vi "rsidr_core_global.vi"() -> ()   [LabVIEW 2020, in "Rohde&Schwarz RTx Oscilloscopes.lvlib"] (continued)
"Descriptive Name"="Protocol SPI Frame Data MOSI", "Data Type"=2, "Command"="BUS{SerialBus}:SPI:FRAM<Frame>:DATA:MOSI?", "Access"=0, "Range Table"="", "Read Callback"="rsrtx_FormatSPIFrameRepCapString_ReadCallback.vi", "Write Callback"="", "Supported Models"="", "Instrument Options"="", "Flags"=0, "Help"="Returns the data words of the specified frame of the MOSI line.\n\nAvailable Repeated Capabilities:\nSerialBus: SB1, SB2, SB3, SB4\r\n\nRemote-control command(s):\nBUS<b>:SPI:FRAMe<n>:DATA:MOSI?"}, {"Level"=3, "Class Only"=FALSE, "Identifier"="RSRTX_ATTR_PROTOCOL_SPI_FRAME_DATA_MISO", "Descriptive Name"="Protocol SPI Frame Data MISO", "Data Type"=2, "Command"="BUS{SerialBus}:SPI:FRAM<Frame>:DATA:MISO?", "Access"=0, "Range Table"="", "Read Callback"="rsrtx_FormatSPIFrameRepCapString_ReadCallback.vi", "Write Callback"="", "Supported Models"="", "Instrument Options"="", "Flags"=0, "Help"="Returns the data words of the specified frame of the MISO line.\n\nAvailable Repeated Capabilities:\nSerialBus: SB1, SB2, SB3, SB4\r\n\nRemote-control command(s):\nBUS<b>:SPI:FRAMe<n>:DATA:MISO?"}, {"Level"=3, "Class Only"=FALSE, "Identifier"="RSRTX_ATTR_PROTOCOL_SPI_WORD_COUNT", "Descriptive Name"="Protocol SPI Word Count", "Data Type"=0, "Command"="BUS{SerialBus}:SPI:FRAM<Frame>:WCO?", "Access"=0, "Range Table"="", "Read Callback"="rsrtx_FormatSPIFrameRepCapInt_ReadCallback.vi", "Write Callback"="", "Supported Models"="", "Instrument Options"="", "Flags"=0, "Help"="Returns the number of words in the specified frame.\n\nAvailable Repeated Capabilities:\nSerialBus: SB1, SB2, SB3, SB4\r\n\nRemote-control command(s):\nBUS<b>:SPI:FRAMe<n>:WCOunt?"}, {"Level"=3, "Class Only"=FALSE, "Identifier"="RSRTX_ATTR_PROTOCOL_SPI_SELECTED_WORD", "Descriptive Name"="Protocol SPI Selected Word", "Data Type"=0, "Command"="", "Access"=2, "Range Table"="", "Read Callback"="", "Write Callback"="", "Supported Models"="", "Instrument Options"="", "Flags"=0, "Help"="Sets selector repeated capability Word.\n\nAvailable Repeated Capabilities:\nNone\n\nRemote-control command(s):\n"}, {"Level"=3, "Class Only"=FALSE, "Identifier"="RSRTX_ATTR_PROTOCOL_SPI_WORD_START", "Descriptive Name"="Protocol SPI Word Start", "Data Type"=1, "Command"="BUS{SerialBus}:SPI:FRAM<Frame>:WORD<Word>:STAR?", "Access"=0, "Range Table"="", "Read Callback"="rsrtx_FormatSPIFrameWordRepCapReal_ReadCallback.vi", "Write Callback"="", "Supported Models"="", "Instrument Options"="", "Flags"=0, "Help"="Returns the start time of the specified data word.\n\nAvailable Repeated Capabilities:\nSerialBus: SB1, SB2, SB3, SB4\r\n\nRemote-control command(s):\nBUS<b>:SPI:FRAMe<n>:WORD<o>:STARt?"}, {"Level"=3, "Class Only"=FALSE, "Identifier"="RSRTX_ATTR_PROTOCOL_SPI_WORD_END", "Descriptive Name"="Protocol SPI Word End", "Data Type"=1, "Command"="BUS{SerialBus}:SPI:FRAM<Frame>:WORD<Word>:STOP?", "Access"=0, "Range Table"="", "Read Callback"="rsrtx_FormatSPIFrameWordRepCapReal_ReadCallback.vi", "Write Callback"="", "Supported Models"="", "Instrument Options"="", "Flags"=0, "Help"="Returns the end time of the specified data word.\n\nAvailable Repeated Capabilities:\nSerialBus: SB1, SB2, SB3, SB4\r\n\nRemote-control command(s):\nBUS<b>:SPI:FRAMe<n>:WORD<o>:STOP?"}, {"Level"=3, "Class Only"=FALSE, "Identifier"="RSRTX_ATTR_PROTOCOL_SPI_WORD_MOSI", "Descriptive Name"="Protocol SPI Word MOSI", "Data Type"=0, "Command"="BUS{SerialBus}:SPI:FRAM<Frame>:WORD<Word>:MOSI?", "Access"=0, "Range Table"="", "Read Callback"="rsrtx_FormatSPIFrameWordRepCapInt_ReadCallback.vi", "Write Callback"="", "Supported Models"="", "Instrument Options"="", "Flags"=0, "Help"="Returns the data value of the specified word on the MOSI line.\nUse this command if only one line is defined.\n\nAvailable Repeated Capabilities:\nSerialBus: SB1, SB2, SB3, SB4\r\n\nRemote-control command(s):\nBUS<b>:SPI:FRAMe<n>:WORD<o>:MOSI?"}, {"Level"=3, "Class Only"=FALSE, "Identifier"="RSRTX_ATTR_PROTOCOL_SPI_WORD_MISO", "Descriptive Name"="Protocol SPI Word MISO", "Data Type"=0, "Command"="BUS{SerialBus}:SPI:FRAM<Frame>:WORD<Word>:MISO?", "Access"=0, "Range Table"="", "Read Callback"="rsrtx_FormatSPIFrameWordRepCapInt_ReadCallback.vi", "Write Callback"="", "Supported Models"="", "Instrument Options"="", "Flags"=0, "Help"="Returns the data value of the specified word on the MISO line.\n\nAvailable Repeated Capabilities:\nSerialBus: SB1, SB2, SB3, SB4\r\n\nRemote-control command(s):\nBUS<b>:SPI:FRAMe<n>:WORD<o>:MISO?"}, {"Level"=3, "Class Only"=TRUE, "Identifier"="", "Descriptive Name"="SSPI", "Data Type"=0, "Command"="", "Access"=0, "Range Table"="", "Read Callback"="", "Write Callback"="", "Supported Models"="", "Instrument Options"="", "Flags"=0, "Help"="SSPI Protocol settings."}, {"Level"=4, "Class Only"=FALSE, "Identifier"="RSRTX_ATTR_PROTOCOL_SSPI_CLOCK_SOURCE", "Descriptive Name"="Protocol SSPI Clock Source", "Data Type"=0, "Command"="BUS{SerialBus}:SSPI:CLOC:SOUR", "Access"=2, "Range Table"="RsRtx_rngChannelAndDigitalSource", "Read Callback"="", "Write Callback"="", "Supported Models"="", "Instrument Options"="", "Flags"=0, "Help"="Sets the input channel for the clock lines.\n\nAvailable Repeated Capabilities:\nSerialBus: SB1, SB2, SB3, SB4\r\n\nRemote-control command(s):\nBUS<b>:SSPI:CLOCk:SOURce"}, {"Level"=4, "Class Only"=FALSE, "Identifier"="RSRTX_ATTR_PROTOCOL_SSPI_DATA_SOURCE", "Descriptive Name"="Protocol SSPI Data Source", "Data Type"=0, "Command"="BUS{SerialBus}:SSPI:DATA:SOUR", "Access"=2, "Range Table"="rsrtx_rngMOSISource", "Read Callback"="", "Write Callback"="", "Supported Models"="", "Instrument Options"="", "Flags"=0, "Help"="Sets the input channel for the clock lines.\n\nAvailable Repeated Capabilities:\nSerialBus: SB1, SB2, SB3, SB4\r\n\nRemote-control command(s):\nBUS<b>:SSPI:DATA:SOURce"}, {"Level"=4, "Class Only"=FALSE, "Identifier"="RSRTX_ATTR_PROTOCOL_SSPI_MISO_SOURCE", "Descriptive Name"="Protocol SSPI MISO Source", "Data Type"=0, "Command"="BUS{SerialBus}:SSPI:MISO:SOUR", "Access"=2, "Range Table"="rsrtx_rngMISOSource", "Read Callback"="", "Write Callback"="", "Supported Models"="", "Instrument Options"="", "Flags"=0, "Help"="Selects the input channel of the optional MISO line.\n\nAvailable Repeated Capabilities:\nSerialBus: SB1, SB2, SB3, SB4\r\n\nRemote-control command(s):\nBUS<b>:SSPI:MISO:SOURce"}, {"Level"=4, "Class Only"=FALSE, "Identifier"="RSRTX_ATTR_PROTOCOL_SSPI_CLOCK_POLARITY", "Descriptive Name"="Protocol SSPI Clock Polarity", "Data Type"=0, "Command"="BUS{SerialBus}:SSPI:CLOC:POL", "Access"=2, "Range Table"="rsrtx_rngPolarity", "Read Callback"="", "Write Callback"="", "Supported Models"="", "Instrument Options"="", "Flags"=0, "Help"="Selects whether transmitted data is high active (high = 1, Positive) or low active (low = 1, Negative).\n\nAvailable Repeated Capabilities:\nSerialBus: SB1, SB2, SB3, SB4\r\n\nRemote-control command(s):\nBUS<b>:SSPI:CLOCk:POLarity"}, {"Level"=4, "Class Only"=FALSE, "Identifier"="RSRTX_ATTR_PROTOCOL_SSPI_DATA_POLARITY", "Descriptive Name"="Protocol SSPI Data Polarity", "Data Type"=0, "Command"="BUS{SerialBus}:SSPI:DATA:POL", "Access"=2, "Range Table"="rsrtx_rngPolarity", "Read Callback"="", "Write Callback"="", "Supported Models"="", "Instrument Options"="", "Flags"=0, "Help"="Selects whether transmitted data is high active (high = 1, Positive) or low active (low = 1, Negative).\n\nAvailable Repeated Capabilities:\nSerialBus: SB1, SB2, SB3, SB4\r\n\nRemote-control command(s):\nBUS<b>:SSPI:DATA:POLarity"}, {"Level"=4, "Class Only"=FALSE, "Identifier"="RSRTX_ATTR_PROTOCOL_SSPI_INTERFRAME_TIME", "Descriptive Name"="Protocol SSPI Interframe Time", "Data Type"=1, "Command"="BUS{SerialBus}:SSPI:BIT", "Access"=2, "Range Table"="rsrtx_rngProtocolBurstIdleTime", "Read Callback"="", "Write Callback"="", "Supported Models"="", "Instrument Options"="", "Flags"=0, "Help"="Within the idle time the data and clock lines are low. A new frame begins when the idle time has expired and the clock line has been inactive during that time. If the time interval between the data words is shorter than the idle time, the words are part of the same frame.\n\nAvailable Repeated Capabilities:\nSerialBus: SB1, SB2, SB3, SB4\r\n\nRemote-control command(s):\nBUS<b>:SSPI:BITime"}, {"Level"=4, "Class Only"=FALSE, "Identifier"="RSRTX_ATTR_PROTOCOL_SSPI_BIT_ORDER", "Descriptive Name"="Protocol SSPI Bit Order", "Data Type"=0, "Command"="BUS{SerialBus}:SSPI:BORD", "Access"=2, "Range Table"="rsrtx_rngProtocolSPIBitOrder", "Read Callback"="", "Write Callback"="", "Supported Models"="", "Instrument Options"="", "Flags"=0, "Help"="Defines if the data of the messages starts with MSB (most significant bit) or LSB (least significant bit).\n\nAvailable Repeated Capabilities:\nSerialBus: SB1, SB2, SB3, SB4\r\n\nRemote-control command(s):\nBUS<b>:SSPI:BORDer"}, {"Level"=4, "Class Only"=FALSE, "Identifier"="RSRTX_ATTR_PROTOCOL_SSPI_WORD_LENGTH", "Descriptive Name"="Protocol SSPI Word Length", "Data Type"=0, "Command"="BUS{SerialBus}:SSPI:SSIZ", "Access"=2, "Range Table"="rsrtx_rngProtocolSPIWordLength", "Read Callback"="", "Write Callback"="", "Supported Models"="", "Instrument Options"="", "Flags"=0, "Help"="Sets the word length, the number of bits in a message.\n\nAvailable Repeated Capabilities:\nSerialBus: SB1, SB2, SB3, SB4\r\n\nRemote-control command(s):\nBUS<b>:SSPI:SSIZe"}, {"Level"=4, "Class Only"=FALSE, "Identifier"="RSRTX_ATTR_PROTOCOL_SSPI_MOSI_POLARITY", "Descriptive Name"="Protocol SSPI MOSI Polarity", "Data Type"=0, "Command"="BUS{SerialBus}:SSPI:MOSI:POL", "Access"=2, "Range Table"="rsrtx_rngProtocolSPIMISOPolarity", "Read Callback"="", "Write Callback"="", "Supported Models"="", "Instrument Options"="", "Flags"=0, "Help"="Selects if transmitted data is high active (high = 1) or low active (low = 1) on the MOSI/MISO line.\n\nAvailable Repeated Capabilities:\nSerialBus: SB1, SB2, SB3, SB4\r\n\nRemote-control command(s):\nBUS<b>:SSPI:MOSI:POLarity"}, {"Level"=4, "Class Only"=FALSE, "Identifier"="RSRTX_ATTR_PROTOCOL_SSPI_MISO_POLARITY", "Descriptive Name"="Protocol SSPI MISO Polarity", "Data Type"=0, "Command"="BUS{SerialBus}:SSPI:MISO:POL", "Access"=2, "Range Table"="rsrtx_rngProtocolSPIMISOPolarity", "Read Callback"="", "Write Callback"="", "Supported Models"="", "Instrument Options"="", "Flags"=0, "Help"="Selects whether transmitted data is high active (high = 1) or low active (low = 1) on the MISO line.\n\nAvailable Repeated Capabilities:\nSerialBus: SB1, SB2, SB3, SB4\r\n\nRemote-control command(s):\nBUS<b>:SSPI:MISO:POLarity"}, {"Level"=2, "Class Only"=TRUE, "Identifier"="", "Descriptive Name"="UART", "Data Type"=0, "Command"="", "Access"=0, "Range Table"="", "Read Callback"="", "Write Callback"="", "Supported Models"="", "Instrument Options"="", "Flags"=0, "Help"="UART/RS232 (EIA-232 serial interface) - decoding requires option K2"}, {"Level"=3, "Class Only"=FALSE, "Identifier"="RSRTX_ATTR_PROTOCOL_UART_SOURCE", "Descriptive Name"="Protocol UART Source", "Data Type"=0, "Command"="BUS{SerialBus}:UART:DATA:SOUR", "Access"=2, "Range Table"="rsrtx_rngUARTSource", "Read Callback"="", "Write Callback"="", "Supported Models"="", "Instrument Options"="", "Flags"=0, "Help"="Selects the input channel of the UART signal.\n\nAvailable Repeated Capabilities:\nSerialBus: SB1, SB2, SB3, SB4\r\n\nRemote-control command(s):\nBUS<b>:UART:DATA:SOURce"}, {"Level"=3, "Class Only"=FALSE, "Identifier"="RSRTX_ATTR_PROTOCOL_UART_RX_SOURCE_LINE", "Descriptive Name"="Protocol UART RX Source Line", "Data Type"=0, "Command"="BUS{SerialBus}:UART:RX:SOUR", "Access"=2, "Range Table"="rsrtx_rngUARTSource", "Read Callback"="", "Write Callback"="", "Supported Models"="", "Instrument Options"="K2", "Flags"=0, "Help"="Selects the input channel of the UART signal.\n\nAvailable Repeated Capabilities:\nSerialBus: SB1, SB2, SB3, SB4\r\n\nRemote-control command(s):\nBUS<b>:UART:RX:SOURce"}, {"Level"=3, "Class Only"=FALSE, "Identifier"="RSRTX_ATTR_PROTOCOL_UART_TX_SOURCE_LINE", "Descriptive Name"="Protocol UART TX Source Line", "Data Type"=0, "Command"="BUS{SerialBus}:UART:TX:SOUR", "Access"=2, "Range Table"="rsrtx_rngUARTTxSource", "Read Callback"="", "Write Callback"="", "Supported Models"="", "Instrument Options"="K2", "Flags"=0, "Help"="Selects the input channel of the UART signal.\n\nAvailable Repeated Capabilities:\nSerialBus: SB1, SB2, SB3, SB4\r\n\nRemote-control command(s):\nBUS<b>:UART:TX:SOURce"}, {"Level"=3, "Class Only"=FALSE, "Identifier"="RSRTX_ATTR_PROTOCOL_UART_POLARITY", "Descriptive Name"="Protocol UART Polarity", "Data Type"=0, "Command"="BUS{SerialBus}:UART:DATA:POL", "Access"=2, "Range Table"="rsrtx_rngPolarity", "Read Callback"="", "Write Callback"="", "Supported Models"="", "Instrument Options"="", "Flags"=0, "Help"="Selects whether transmitted data is high active (high = 1, Positive) or low active (low = 1, Negative). Alternative Command for RSRTX_ATTR_PROTOCOL_UART_IDLE_STATE_POLARITY.\n\nAvailable Repeated Capabilities:\nSerialBus: SB1, SB2, SB3, SB4\r\n\nRemote-control command(s):\nBUS<b>:UART:DATA:POLarity"}, {"Level"=3, "Class Only"=FALSE, "Identifier"="RSRTX_ATTR_PROTOCOL_UART_IDLE_STATE_POLARITY", "Descriptive Name"="Protocol UART Idle State Polarity", "Data Type"=0, "Command"="BUS{SerialBus}:UART:POL", "Access"=2, "Range Table"="RsRtx_rngIdleStatePolarity", "Read Callback"="", "Write Callback"="", "Supported Models"="", "Instrument Options"="", "Flags"=0, "Help"="Defines the logic levels of the bus. The idle state corresponds to a logic 1, and the start bit to a logic 0.\nAlternative command for RSRTX_ATTR_PROTOCOL_UART_POLARITY\n\nAvailable Repeated Capabilities:\nSerialBus: SB1, SB2, SB3, SB4\r\n\nRemote-control command(s):\nBUS<b>:UART:POLarity"}, {"Level"=3, "Class Only"=FALSE, "Identifier"="RSRTX_ATTR_PROTOCOL_UART_INTERFRAME_TIME", "Descriptive Name"="Protocol UART Interframe Time", "Data Type"=1, "Command"="BUS{SerialBus}:UART:BIT", "Access"=2, "Range Table"="", "Read Callback"="", "Write Callback"="", "Supported Models"="", "Instrument Options"="", "Flags"=0, "Help"="Sets the minimal time between two data frames (packets), that is, between the last stop bit and the start bit of the next frame.\n\nAvailable Repeated Capabilities:\nSerialBus: SB1, SB2, SB3, SB4\r\n\nRemote-control command(s):\nBUS<b>:UART:BITime"}, {"Level"=3, "Class Only"=FALSE, "Identifier"="RSRTX_ATTR_PROTOCOL_UART_WORD_LENGTH", "Descriptive Name"="Protocol UART Word Length", "Data Type"=0, "Command"="BUS{SerialBus}:UART:SSIZ", "Access"=2, "Range Table"="rsrtx_rngProtocolUARTWordLength", "Read Callback"="", "Write Callback"="", "Supported Models"="", "Instrument Options"="", "Flags"=0, "Help"="Sets the number of data bits in a message.\n\nAvailable Repeated Capabilities:\nSerialBus: SB1, SB2, SB3, SB4\r\n\nRemote-control command(s):\nBUS<b>:UART:SSIZe"}, {"Level"=3, "Class Only"=FALSE, "Identifier"="RSRTX_ATTR_PROTOCOL_UART_BIT_RATE", "Descriptive Name"="Protocol UART Bit Rate", "Data Type"=1, "Command"="BUS{SerialBus}:UART:BAUD", "Access"=2, "Range Table"="rsrtx_rngProtocolUARTBitRate", "Read Callback"="", "Write Callback"="", "Supported Models"="", "Instrument Options"="", "Flags"=0, "Help"="Sets the number of transmitted bits per second.\n\nAvailable Repeated Capabilities:\nSerialBus: SB1, SB2, SB3, SB4\r\n\nRemote-control command(s):\nBUS<b>:UART:BAUDrate"}, {"Level"=3, "Class Only"=FALSE, "Identifier"="RSRTX_ATTR_PROTOCOL_UART_PARITY", "Descriptive Name"="Protocol UART Parity", "Data Type"=0, "Command"="BUS{SerialBus}:UART:PAR", "Access"=2, "Range Table"="rsrtx_rngProtocolUARTParity", "Read Callback"="", "Write Callback"="", "Supported Models"="", "Instrument Options"="", "Flags"=0, "Help"="Defines the optional parity bit that is used for error detection.\n\nAvailable Repeated Capabilities:\nSerialBus: SB1, SB2, SB3, SB4\r\n\nRemote-control command(s):\nBUS<b>:UART:PARity"}, {"Level"=3, "Class Only"=FALSE, "Identifier"="RSRTX_ATTR_PROTOCOL_UART_STOP_BITS", "Descriptive Name"="Protocol UART Stop Bits", "Data Type"=0, "Command"="BUS{SerialBus}:UART:SBIT", "Access"=2, "Range Table"="rsrtx_rngProtocolUARTStopBits", "Read Callback"="", "Write Callback"="", "Supported Models"="", "Instrument Options"="", "Flags"=0, "Help"="Sets the stop bits.\n\nAvailable Repeated Capabilities:\nSerialBus: SB1, SB2, SB3, SB4\r\n\nRemote-control command(s):\nBUS<b>:UART:SBIT"}, {"Level"=3, "Class Only"=FALSE, "Identifier"="RSRTX_ATTR_PROTOCOL_UART_FRAME_COUNT", "Descriptive Name"="Protocol UART Frame Count", "Data Type"=0, "Command"="BUS{SerialBus}:UART:FCO?", "Access"=0, "Range Table"="", "Read Callback"="", "Write Callback"="", "Supported Models"="", "Instrument Options"="K2", "Flags"=0, "Help"="Return the number of decoded frames on the data line.\n\nAvailable Repeated Capabilities:\nSerialBus: SB1, SB2, SB3, SB4\r\n\nRemote-control command(s):\nBUS<b>:UART:FCOunt?"}, {"Level"=3, "Class Only"=FALSE, "Identifier"="RSRTX_ATTR_PROTOCOL_UART_RX_FRAME_COUNT", "Descriptive Name"="Protocol UART RX Frame Count", "Data Type"=0, "Command"="BUS{SerialBus}:UART:RX:FCO?", "Access"=0, "Range Table"="", "Read Callback"="", "Write Callback"="", "Supported Models"="", "Instrument Options"="K2", "Flags"=0, "Help"="Queries the number of decoded frames on the RX lines, respectivley.\n\nAvailable Repeated Capabilities:\nSerialBus: SB1, SB2, SB3, SB4\r\n\nRemote-control command(s):\nBUS<b>:UART:RX:FCOunt?"}, {"Level"=3, "Class Only"=FALSE, "Identifier"="RSRTX_ATTR_PROTOCOL_UART_TX_FRAME_COUNT", "Descriptive Name"="Protocol UART TX Frame Count", "Data Type"=0, "Command"="BUS{SerialBus}:UART:TX:FCO?", "Access"=0, "Range Table"="", "Read Callback"="", "Write Callback"="", "Supported Models"="", "Instrument Options"="K2", "Flags"=0, "Help"="Queries the number of decoded frames on the TX lines, respectivley.\n\nAvailable Repeated Capabilities:\nSerialBus: SB1, SB2, SB3, SB4\r\n\nRemote-control command(s):\nBUS<b>:UART:TX:FCOunt?"}, {"Level"=3, "Class Only"=FALSE, "Identifier"="RSRTX_ATTR_PROTOCOL_UART_SELECTED_FRAME", "Descriptive Name"="Protocol UART Selected Frame", "Data Type"=0, "Command"="", "Access"=2, "Range Table"="", "Read Callback"="", "Write Callback"="", "Supported Models"="", "Instrument Options"="", "Flags"=0, "Help"="Sets selector repeated capability Frame.\n\nAvailable Repeated Capabilities:\nNone\n\nRemote-control command(s):\n"}, {"Level"=3, "Class Only"=FALSE, "Identifier"="RSRTX_ATTR_PROTOCOL_UART_FRAME_STATE", "Descriptive Name"="Protocol UART Frame State", "Data Type"=0, "Command"="BUS{SerialBus}:UART:FRAM<Frame>:STAT?", "Access"=0, "Range Table"="RsRtx_rngUARTFrameState", "Read Callback"="rsrtx_FormatUARTFrameRepCapInt_ReadCallback.vi", "Write Callback"="", "Supported Models"="", "Instrument Options"="K2", "Flags"=0, "Help"="Returns the status of the specified frame.\n\nAvailable Repeated Capabilities:\nSerialBus: SB1, SB2, SB3, SB4\r\n\nRemote-control command(s):\nBUS<b>:UART:FRAMe<n>:STATe?"}, {"Level"=3, "Class Only"=FALSE, "Identifier"="RSRTX_ATTR_PROTOCOL_UART_RX_FRAME_STATE", "Descriptive Name"="Protocol UART Rx Frame State", "Data Type"=0, "Command"="BUS{SerialBus}:UART:RX:FRAM<Frame>:STAT?", "Access"=0, "Range Table"="RsRtx_rngUARTFrameState", "Read Callback"="rsrtx_FormatUARTFrameRepCapInt_ReadCallback.vi", "Write Callback"="", "Supported Models"="", "Instrument Options"="K2", "Flags"=0, "Help"="Returns the status of the specified frame.\n\nAvailable Repeated Capabilities:\nSerialBus: SB1, SB2, SB3, SB4\r\n\nRemote-control command(s):\nBUS<b>:UART:RX:FRAMe<n>:STATe?"}, {"Level"=3, "Class Only"=FALSE, "Identifier"="RSRTX_ATTR_PROTOCOL_UART_TX_FRAME_STATE", "Descriptive Name"="Protocol UART Tx Frame State", "Data Type"=0, "Command"="BUS{SerialBus}:UART:TX:FRAM<Frame>:STAT?", "Access"=0, "Range Table"="RsRtx_rngUARTFrameState", "Read Callback"="rsrtx_FormatUARTFrameRepCapInt_ReadCallback.vi", "Write Callback"="", "Supported Models"="", "Instrument Options"="K2", "Flags"=0, "Help"="Returns the status of the specified frame.\n\nAvailable Repeated Capabilities:\nSerialBus: SB1, SB2, SB3, SB4\r\n\nRemote-control command(s):\nBUS<b>:UART:TX:FRAMe<n>:STATe?"}, {"Level"=3, "Class Only"=FALSE, "Identifier"="RSRTX_ATTR_PROTOCOL_UART_FRAME_START", "Descriptive Name"="Protocol UART Frame Start", "Data Type"=1, "Command"="BUS{SerialBus}:UART:FRAM<Frame>:STAR?", "Access"=0, "Range Table"="", "Read Callback"="rsrtx_FormatUARTFrameRepCapReal_ReadCallback.vi", "Write Callback"="", "Supported Models"="", "Instrument Options"="K2", "Flags"=0, "Help"="Return the start time of the specified frame.\n\nAvailable Repeated Capabilities:\nSerialBus: SB1, SB2, SB3, SB4\r\n\nRemote-control command(s):\nBUS<b>:UART:FRAMe<n>:STARt?"}, {"Level"=3, "Class Only"=FALSE, "Identifier"="RSRTX_ATTR_PROTOCOL_UART_RX_FRAME_START", "Descriptive Name"="Protocol UART Rx Frame Start", "Data Type"=1, "Command"="BUS{SerialBus}:UART:RX:FRAM<Frame>:STAR?", "Access"=0, "Range Table"="", "Read Callback"="rsrtx_FormatUARTFrameRepCapReal_ReadCallback.vi", "Write Callback"="", "Supported Models"="", "Instrument Options"="K2", "Flags"=0, "Help"="Return the start time of the specified frame.\n\nAvailable Repeated Capabilities:\nSerialBus: SB1, SB2, SB3, SB4\r\n\nRemote-control command(s):\nBUS<b>:UART:RX:FRAMe<n>:STARt?"}, {"Level"=3, "Class Only"=FALSE, "Identifier"="RSRTX_ATTR_PROTOCOL_UART_TX_FRAME_START", "Descriptive Name"="Protocol UART Tx Frame Start", "Data Type"=1, "Command"="BUS{SerialBus}:UART:TX:FRAM<Frame>:STAR?", "Access"=0, "Range Table"="", "Read Callback"="rsrtx_FormatUARTFrameRepCapReal_ReadCallback.vi", "Write Callback"="", "Supported Models"="", "Instrument Options"="K2", "Flags"=0, "Help"="Return the start time of the specified frame.\n\nAvailable Repeated Capabilities:\nSerialBus: SB1, SB2, SB3, SB4\r\n\nRemote-control command(s):\nBUS<b>:UART:TX:FRAMe<n>:STARt?"}, {"Level"=3, "Class Only"=FALSE, "Identifier"="RSRTX_ATTR_PROTOCOL_UART_FRAME_END", "Descriptive Name"="Protocol UART Frame End", "Data Type"=1, "Command"="BUS{SerialBus}:UART:FRAM<Frame>:STOP?", "Access"=0, "Range Table"="", "Read Callback"="rsrtx_FormatUARTFrameRepCapReal_ReadCallback.vi", "Write Callback"="", "Supported Models"="", "Instrument Options"="K2", "Flags"=0, "Help"="Return the end time of the specified frame.\n\nAvailable Repeated Capabilities:\nSerialBus: SB1, SB2, SB3, SB4\r\n\nRemote-control command(s):\nBUS<b>:UART:FRAMe<n>:STOP?"}, {"Level"=3, "Class Only"=FALSE, "Identifier"="RSRTX_ATTR_PROTOCOL_UART_RX_FRAME_END", "Descriptive Name"="Protocol UART Rx Frame End", "Data Type"=1, "Command"="BUS{SerialBus}:UART:RX:FRAM<Frame>:STOP?", "Access"=0, "Range Table"="", "Read Callback"="rsrtx_FormatUARTFrameRepCapReal_ReadCallback.vi", "Write Callback"="", "Supported Models"="", "Instrument Options"="K2", "Flags"=0, "Help"="Return the end time of the specified frame.\n\nAvailable Repeated Capabilities:\nSerialBus: SB1, SB2, SB3, SB4\r\n\nRemote-control command(s):\nBUS<b>:UART:RX:FRAMe<n>:STOP?"}, {"Level"=3, "Class Only"=FALSE, "Identifier"="RSRTX_ATTR_PROTOCOL_UART_TX_FRAME_END", "Descriptive Name"="Protocol UART Tx Frame End", "Data Type"=1, "Command"="BUS{SerialBus}:UART:TX:FRAM<Frame>:STOP?", "Access"=0, "Range Table"="", "Read Callback"="rsrtx_FormatUARTFrameRepCapReal_ReadCallback.vi", "Write Callback"="", "Supported Models"="", "Instrument Options"="K2", "Flags"=0, "Help"="Return the end time of the specified frame.\n\nAvailable Repeated Capabilities:\nSerialBus: SB1, SB2, SB3, SB4\r\n\nRemote-control command(s):\nBUS<b>:UART:TX:FRAMe<n>:STOP?"}, {"Level"=3, "Class Only"=FALSE, "Identifier"="RSRTX_ATTR_PROTOCOL_UART_WORD_COUNT", "Descriptive Name"="Protocol UART Word Count", "Data Type"=0, "Command"="BUS{SerialBus}:UART:FRAM<Frame>:WCO?", "Access"=0, "Range Table"="", "Read Callback"="rsrtx_FormatUARTFrameRepCapInt_ReadCallback.vi", "Write Callback"="", "Supported Models"="", "Instrument Options"="", "Flags"=0, "Help"="Returns the number of words in the specified frame.\n\nAvailable Repeated Capabilities:\nSerialBus: SB1, SB2, SB3, SB4\r\n\nRemote-control command(s):\nBUS<b>:UART:FRAMe<n>:WCOunt?"}, {"Level"=3, "Class Only"=FALSE, "Identifier"="RSRTX_ATTR_PROTOCOL_UART_RX_WORD_COUNT", "Descriptive Name"="Protocol UART Rx Word Count", "Data Type"=0, "Command"="BUS{SerialBus}:UART:RX:FRAM<Frame>:WCO?", "Access"=0, "Range Table"="", "Read Callback"="rsrtx_FormatUARTFrameRepCapInt_ReadCallback.vi", "Write Callback"="", "Supported Models"="", "Instrument Options"="", "Flags"=0, "Help"="Returns the number of words in the specified frame.\n\nAvailable Repeated Capabilities:\nSerialBus: SB1, SB2, SB3, SB4\r\n\nRemote-control command(s):\nBUS<b>:UART:RX:FRAMe<n>:WCOunt?"}, {"Level"=3, "Class Only"=FALSE, "Identifier"="RSRTX_ATTR_PROTOCOL_UART_TX_WORD_COUNT", "Descriptive Name"="Protocol UART Tx Word Count", "Data Type"=0, "Command"="BUS{SerialBus}:UART:TX:FRAM<Frame>:WCO?", "Access"=0, "Range Table"="", "Read Callback"="rsrtx_FormatUARTFrameRepCapInt_ReadCallback.vi", "Write Callback"="", "Supported Models"="", "Instrument Options"="", "Flags"=0, "Help"="Returns the number of words in the specified frame.\n\nAvailable Repeated Capabilities:\nSerialBus: SB1, SB2, SB3, SB4\r\n\nRemote-control command(s):\nBUS<b>:UART:TX:FRAMe<n>:WCOunt?"}, {"Level"=3, "Class Only"=FALSE, "Identifier"="RSRTX_ATTR_PROTOCOL_UART_SELECTED_WORD", "Descriptive Name"="Protocol UART Selected Word", "Data Type"=0, "Command"="", "Access"=2, "Range Table"="", "Read Callback"="", "Write Callback"="", "Supported Models"="", "Instrument Options"="", "Flags"=0, "Help"="Sets selector repeated capability Word.\n\nAvailable Repeated Capabilities:\nNone\n\nRemote-control command(s):\n"}, {"Level"=3, "Class Only"=FALSE, "Identifier"="RSRTX_ATTR_PROTOCOL_UART_WORD_VALUE", "Descriptive Name"="Protocol UART Word Value", "Data Type"=0, "Command"="BUS{SerialBus}:UART:FRAM<Frame>:WORD<Word>:VAL?", "Access"=0, "Range Table"="", "Read Callback"="rsrtx_FormatUARTFrameWordRepCapInt_ReadCallback.vi", "Write Callback"="", "Supported Models"="", "Instrument Options"="", "Flags"=0, "Help"="Returns the value of words in the specified frame.\n\nAvailable Repeated Capabilities:\nSerialBus: SB1, SB2, SB3, SB4\r\n\nRemote-control command(s):\nBUS<b>:UART:FRAMe<n>:WORD<o>:VALue?"}, {"Level"=3, "Class Only"=FALSE, "Identifier"="RSRTX_ATTR_PROTOCOL_UART_RX_WORD_VALUE", "Descriptive Name"="Protocol UART Rx Word Value", "Data Type"=0, "Command"="BUS{SerialBus}:UART:RX:FRAM<Frame>:WORD<Word>:VAL?", "Access"=0, "Range Table"="", "Read Callback"="rsrtx_FormatUARTFrameWordRepCapInt_ReadCallback.vi", "Write Callback"="", "Supported Models"="", "Instrument Options"="", "Flags"=0, "Help"="Returns the value of words in the specified frame.\n\nAvailable Repeated Capabilities:\nSerialBus: SB1, SB2, SB3, SB4\r\n\nRemote-control command(s):\nBUS<b>:UART:RX:FRAMe<n>:WORD<o>:VALue?"}, {"Level"=3, "Class Only"=FALSE, "Identifier"="RSRTX_ATTR_PROTOCOL_UART_TX_WORD_VALUE", "Descriptive Name"="Protocol UART Tx Word Value", "Data Type"=0, "Command"="BUS{SerialBus}:UART:TX:FRAM<Frame>:WORD<Word>:VAL?", "Access"=0, "Range Table"="", "Read Callback"="rsrtx_FormatUARTFrameWordRepCapInt_ReadCallback.vi", "Write Callback"="", "Supported Models"="", "Instrument Options"="", "Flags"=0, "Help"="Returns the value of words in the specified frame.\n\nAvailable Repeated Capabilities:\nSerialBus: SB1, SB2, SB3, SB4\r\n\nRemote-control command(s):\nBUS<b>:UART:TX:FRAMe<n>:WORD<o>:VALue?"}, {"Level"=3, "Class Only"=FALSE, "Identifier"="RSRTX_ATTR_PROTOCOL_UART_WORD_START", "Descriptive Name"="Protocol UART Word Start", "Data Type"=1, "Command"="BUS{SerialBus}:UART:FRAM<Frame>:WORD<Word>:STAR?", "Access"=0, "Range Table"="", "Read Callback"="rsrtx_FormatUARTFrameWordRepCapReal_ReadCallback.vi", "Write Callback"="", "Supported Models"="", "Instrument Options"="K2", "Flags"=0, "Help"="Returns the start time of words in the specified frame.\n\nAvailable Repeated Capabilities:\nSerialBus: SB1, SB2, SB3, SB4\r\n\nRemote-control command(s):\nBUS<b>:UART:FRAMe<n>:WORD<o>:STARt?"}, {"Level"=3, "Class Only"=FALSE, "Identifier"="RSRTX_ATTR_PROTOCOL_UART_RX_WORD_START", "Descriptive Name"="Protocol UART Rx Word Start", "Data Type"=1, "Command"="BUS{SerialBus}:UART:RX:FRAM<Frame>:WORD<Word>:STAR?", "Access"=0, "Range Table"="", "Read Callback"="rsrtx_FormatUARTFrameWordRepCapReal_ReadCallback.vi", "Write Callback"="", "Supported Models"="", "Instrument Options"="K2", "Flags"=0, "Help"="Returns the start time of words in the specified frame.\n\nAvailable Repeated Capabilities:\nSerialBus: SB1, SB2, SB3, SB4\r\n\nRemote-control command(s):\nBUS<b>:UART:RX:FRAMe<n>:WORD<o>:STARt?"}, {"Level"=3, "Class Only"=FALSE, "Identifier"="RSRTX_ATTR_PROTOCOL_UART_TX_WORD_START", "Descriptive Name"="Protocol UART Tx Word Start", "Data Type"=1, "Command"="BUS{SerialBus}:UART:TX:FRAM<Frame>:WORD<Word>:STAR?", "Access"=0, "Range Table"="", "Read Callback"="rsrtx_FormatUARTFrameWordRepCapReal_ReadCallback.vi", "Write Callback"="", "Supported Models"="", "Instrument Options"="K2", "Flags"=0, "Help"="Returns the start time of words in the specified frame.\n\nAvailable Repeated Capabilities:\nSerialBus: SB1, SB2, SB3, SB4\r\n\nRemote-control command(s):\nBUS<b>:UART:TX:FRAMe<n>:WORD<o>:STARt?"}, {"Level"=3, "Class Only"=FALSE, "Identifier"="RSRTX_ATTR_PROTOCOL_UART_WORD_END", "Descriptive Name"="Protocol UART Word End", "Data Type"=1, "Command"="BUS{SerialBus}:UART:FRAM<Frame>:WORD<Word>:STOP?", "Access"=0, "Range Table"="", "Read Callback"="rsrtx_FormatUARTFrameWordRepCapReal_ReadCallback.vi", "Write Callback"="", "Supported Models"="", "Instrument Options"="K2", "Flags"=0, "Help"="Returns the end time of words in the specified frame.\n\nAvailable Repeated Capabilities:\nSerialBus: SB1, SB2, SB3, SB4\r\n\nRemote-control command(s):\nBUS<b>:UART:FRAMe<n>:WORD<o>:STOP?"}, {"Level"=3, "Class Only"=FALSE, "Identifier"="RSRTX_ATTR_PROTOCOL_UART_RX_WORD_END", "Descriptive Name"="Protocol UART Rx Word End", "Data Type"=1, "Command"="BUS{SerialBus}:UART:RX:FRAM<Frame>:WORD<Word>:STOP?", "Access"=0, "Range Table"="", "Read Callback"="rsrtx_FormatUARTFrameWordRepCapReal_ReadCallback.vi", "Write Callback"="", "Supported Models"="", "Instrument Options"="K2", "Flags"=0, "Help"="Returns the end time of words in the specified frame.\n\nAvailable Repeated Capabilities:\nSerialBus: SB1, SB2, SB3, SB4\r\n\nRemote-control command(s):\nBUS<b>:UART:RX:FRAMe<n>:WORD<o>:STOP?"}, {"Level"=3, "Class Only"=FALSE, "Identifier"="RSRTX_ATTR_PROTOCOL_UART_TX_WORD_END", "Descriptive Name"="Protocol UART Tx Word End", "Data Type"=1, "Command"="BUS{SerialBus}:UART:TX:FRAM<Frame>:WORD<Word>:STOP?", "Access"=0, "Range Table"="", "Read Callback"="rsrtx_FormatUARTFrameWordRepCapReal_ReadCallback.vi", "Write Callback"="", "Supported Models"="", "Instrument Options"="K2", "Flags"=0, "Help"="Returns the end time of words in the specified frame.\n\nAvailable Repeated Capabilities:\nSerialBus: SB1, SB2, SB3, SB4\r\n\nRemote-control command(s):\nBUS<b>:UART:TX:FRAMe<n>:WORD<o>:STOP?"}, {"Level"=3, "Class Only"=FALSE, "Identifier"="RSRTX_ATTR_PROTOCOL_UART_WORD_ENABLED", "Descriptive Name"="Protocol UART Word Enabled", "Data Type"=0, "Command"="BUS{SerialBus}:UART:FRAM<Frame>:WORD<Word>:STAT?", "Access"=0, "Range Table"="rsrtx_rngUARTWordEnabled", "Read Callback"="rsrtx_FormatUARTFrameWordRepCapInt_ReadCallback.vi", "Write Callback"="", "Supported Models"="", "Instrument Options"="", "Flags"=0, "Help"="Returns the state of words in the specified frame.\n\nAvailable Repeated Capabilities:\nSerialBus: SB1, SB2, SB3, SB4\r\n\nRemote-control command(s):\nBUS<b>:UART:FRAMe<n>:WORD<o>:STATe?"}, {"Level"=3, "Class Only"=FALSE, "Identifier"="RSRTX_ATTR_PROTOCOL_UART_RX_WORD_ENABLED", "Descriptive Name"="Protocol UART Rx Word Enabled", "Data Type"=0, "Command"="BUS{SerialBus}:UART:RX:FRAM<Frame>:WORD<Word>:STATe?", "Access"=0, "Range Table"="rsrtx_rngUARTWordEnabled", "Read Callback"="rsrtx_FormatUARTFrameWordRepCapInt_ReadCallback.vi", "Write Callback"="", "Supported Models"="", "Instrument Options"="", "Flags"=0, "Help"="Returns the state of words in the specified frame.\n\nAvailable Repeated Capabilities:\nSerialBus: SB1, SB2, SB3, SB4\r\n\nRemote-control command(s):\nBUS<b>:UART:RX:FRAMe<n>:WORD<o>:STATe?"}, {"Level"=3, "Class Only"=FALSE, "Identifier"="RSRTX_ATTR_PROTOCOL_UART_TX_WORD_ENABLED", "Descriptive Name"="Protocol UART Tx Word Enabled", "Data Type"=0, "Command"="BUS{SerialBus}:UART:TX:FRAM<Frame>:WORD<Word>:STATe?", "Access"=0, "Range Table"="rsrtx_rngUARTWordEnabled", "Read Callback"="rsrtx_FormatUARTFrameWordRepCapInt_ReadCallback.vi", "Write Callback"="", "Supported Models"="", "Instrument Options"="", "Flags"=0, "Help"="Returns the state of words in the specified frame.\n\nAvailable Repeated Capabilities:\nSerialBus: SB1, SB2, SB3, SB4\r\n\nRemote-control command(s):\nBUS<b>:UART:TX:FRAMe<n>:WORD<o>:STATe?"}, {"Level"=3, "Class Only"=FALSE, "Identifier"="RSRTX_ATTR_PROTOCOL_UART_WORD_SOURCE", "Descriptive Name"="Protocol UART Word Source", "Data Type"=0, "Command"="BUS{SerialBus}:UART:FRAM<Frame>:WORD<Word>:SOUR?", "Access"=0, "Range Table"="RsRtx_rngUARTFrameSource", "Read Callback"="rsrtx_FormatUARTFrameWordRepCapInt_ReadCallback.vi", "Write Callback"="", "Supported Models"="", "Instrument Options"="", "Flags"=0, "Help"="Returns the value of word source in the specified frame.\n\nAvailable Repeated Capabilities:\nSerialBus: SB1, SB2, SB3, SB4\r\n\nRemote-control command(s):\nBUS<b>:UART:FRAMe<n>:WORD<o>:SOURce?"}, {"Level"=2, "Class Only"=TRUE, "Identifier"="", "Descriptive Name"="LIN", "Data Type"=0, "Command"="", "Access"=0, "Range Table"="", "Read Callback"="", "Write Callback"="", "Supported Models"="", "Instrument Options"="", "Flags"=0, "Help"="This class contains attributes that configure the LIN (Local Interconnect Network)\n\nAttributes in this class requires option K3."}, {"Level"=3, "Class Only"=FALSE, "Identifier"="RSRTX_ATTR_PROTOCOL_LIN_SOURCE", "Descriptive Name"="Protocol LIN Source", "Data Type"=0, "Command"="BUS{SerialBus}:LIN:DATA:SOUR", "Access"=2, "Range Table"="RsRtx_rngChannelAndDigitalSource", "Read Callback"="", "Write Callback"="", "Supported Models"="", "Instrument Options"="K3", "Flags"=0, "Help"="Configures source waveform of the data line.\n\nAvailable Repeated Capabilities:\nSerialBus: SB1, SB2, SB3, SB4\r\n\nRemote-control command(s):\nBUS<b>:LIN:DATA:SOURce"}, {"Level"=3, "Class Only"=FALSE, "Identifier"="RSRTX_ATTR_PROTOCOL_LIN_POLARITY", "Descriptive Name"="Protocol LIN Polarity", "Data Type"=0, "Command"="BUS{SerialBus}:LIN:POL", "Access"=2, "Range Table"="rsrtx_rngProtocolLINPolarity", "Read Callback"="", "Write Callback"="", "Supported Models"="", "Instrument Options"="", "Flags"=0, "Help"="Selects whether transmitted signal is high active (high = 1) or low active (low= 1).\n\nAvailable Repeated Capabilities:\nSerialBus: SB1, SB2, SB3, SB4\r\n\nRemote-control command(s):\nBUS<b>:LIN:POLarity"}, {"Level"=3, "Class Only"=FALSE, "Identifier"="RSRTX_ATTR_PROTOCOL_LIN_STANDARD", "Descriptive Name"="Protocol LIN Standard", "Data Type"=0, "Command"="BUS{SerialBus}:LIN:STAN", "Access"=2, "Range Table"="rsrtx_rngProtocolLINStandard", "Read Callback"="", "Write Callback"="", "Supported Models"="", "Instrument Options"="K3", "Flags"=0, "Help"="Selects the version of the LIN standard that is used in the DUT. The setting mainly defines the checksum version used during decoding.\n\nAvailable Repeated Capabilities:\nSerialBus: SB1, SB2, SB3, SB4\r\n\nRemote-control command(s):\nBUS<b>:LIN:STANdard"}, {"Level"=3, "Class Only"=FALSE, "Identifier"="RSRTX_ATTR_PROTOCOL_LIN_BIT_RATE", "Descriptive Name"="Protocol LIN Bit Rate", "Data Type"=1, "Command"="BUS{SerialBus}:LIN:BITR", "Access"=2, "Range Table"="", "Read Callback"="", "Write Callback"="", "Supported Models"="", "Instrument Options"="K3", "Flags"=0, "Help"="Sets the number of transmitted bits per second.\n\nAvailable Repeated Capabilities:\nSerialBus: SB1, SB2, SB3, SB4\r\n\nRemote-control command(s):\nBUS<b>:LIN:BITRate"}, {"Level"=3, "Class Only"=FALSE, "Identifier"="RSRTX_ATTR_PROTOCOL_LIN_FRAME_COUNT", "Descriptive Name"="Protocol LIN Frame Count", "Data Type"=0, "Command"="BUS{SerialBus}:LIN:FCO?", "Access"=0, "Range Table"="", "Read Callback"="", "Write Callback"="", "Supported Models"="", "Instrument Options"="K3", "Flags"=0, "Help"="Queries the number of decoded frames.\n\nAvailable Repeated Capabilities:\nSerialBus: SB1, SB2, SB3, SB4\r\n\nRemote-control command(s):\nBUS<b>:LIN:FCOunt?"}, {"Level"=3, "Class Only"=FALSE, "Identifier"="RSRTX_ATTR_PROTOCOL_LIN_SELECTED_FRAME", "Descriptive Name"="Protocol LIN Selected Frame", "Data Type"=0, "Command"="", "Access"=2, "Range Table"="", "Read Callback"="", "Write Callback"="", "Supported Models"="", "Instrument Options"="", "Flags"=0, "Help"="Sets selector repeated capability Frame.\n\nAvailable Repeated Capabilities:\nNone\n\nRemote-control command(s):\n"}, {"Level"=3, "Class Only"=FALSE, "Identifier"="RSRTX_ATTR_PROTOCOL_LIN_FRAME_DATA", "Descriptive Name"="Protocol LIN Frame Data", "Data Type"=2, "Command"="BUS{SerialBus}:LIN:FRAM<Frame>:DATA?", "Access"=0, "Range Table"="", "Read Callback"="rsrtx_FormatLINFrameRepCapString_ReadCallback.vi", "Write Callback"="", "Supported Models"="", "Instrument Options"="", "Flags"=0, "Help"="Returns the data bytes of the specified frame.\n\nAvailable Repeated Capabilities:\nSerialBus: SB1, SB2, SB3, SB4\r\n\nRemote-control command(s):\nBUS<b>:LIN:FRAMe<n>:DATA?"}, {"Level"=3, "Class Only"=FALSE, "Identifier"="RSRTX_ATTR_PROTOCOL_LIN_FRAME_STATUS", "Descriptive Name"="Protocol LIN Frame Status", "Data Type"=0, "Command"="BUS{SerialBus}:LIN:FRAM<Frame>:STAT?", "Access"=0, "Range Table"="rsrtx_rngLINFrameStatus", "Read Callback"="rsrtx_FormatLINFrameRepCapInt_ReadCallback.vi", "Write Callback"="", "Supported Models"="", "Instrument Options"="", "Flags"=0, "Help"="Returns the status of the specified frame.\n\nAvailable Repeated Capabilities:\nSerialBus: SB1, SB2, SB3, SB4\r\n\nRemote-control command(s):\nBUS<b>:LIN:FRAMe<n>:STATus?"}, {"Level"=3, "Class Only"=FALSE, "Identifier"="RSRTX_ATTR_PROTOCOL_LIN_FRAME_START", "Descriptive Name"="Protocol LIN Frame Start", "Data Type"=1, "Command"="BUS{SerialBus}:LIN:FRAM<Frame>:STAR?", "Access"=0, "Range Table"="", "Read Callback"="rsrtx_FormatLINFrameRepCapReal_ReadCallback.vi", "Write Callback"="", "Supported Models"="", "Instrument Options"="", "Flags"=0, "Help"="Returns the start time of the specified frame.\n\nAvailable Repeated Capabilities:\nSerialBus: SB1, SB2, SB3, SB4\r\n\nRemote-control command(s):\nBUS<b>:LIN:FRAMe<n>:STARt?"}, {"Level"=3, "Class Only"=FALSE, "Identifier"="RSRTX_ATTR_PROTOCOL_LIN_FRAME_END", "Descriptive Name"="Protocol LIN Frame End", "Data Type"=1, "Command"="BUS{SerialBus}:LIN:FRAM<Frame>:STOP?", "Access"=0, "Range Table"="", "Read Callback"="rsrtx_FormatLINFrameRepCapReal_ReadCallback.vi", "Write Callback"="", "Supported Models"="", "Instrument Options"="", "Flags"=0, "Help"="Returns the end time of the specified frame.\n\nAvailable Repeated Capabilities:\nSerialBus: SB1, SB2, SB3, SB4\r\n\nRemote-control command(s):\nBUS<b>:LIN:FRAMe<n>:STOP?"}, {"Level"=3, "Class Only"=FALSE, "Identifier"="RSRTX_ATTR_PROTOCOL_LIN_FRAME_CHECKSUM_ENABLED", "Descriptive Name"="Protocol LIN Frame Checksum Enabled", "Data Type"=0, "Command"="BUS{SerialBus}:LIN:FRAM<Frame>:CSST?", "Access"=0, "Range Table"="rsrtx_rngLINChecksum", "Read Callback"="rsrtx_FormatLINFrameRepCapInt_ReadCallback.vi", "Write Callback"="", "Supported Models"="", "Instrument Options"="", "Flags"=0, "Help"="Returns the checksum state of the specified frame.\n\nAvailable Repeated Capabilities:\nSerialBus: SB1, SB2, SB3, SB4\r\n\nRemote-control command(s):\nBUS<b>:LIN:FRAMe<n>:CSSTate?"}, {"Level"=3, "Class Only"=FALSE, "Identifier"="RSRTX_ATTR_PROTOCOL_LIN_FRAME_CHECKSUM_VALUE", "Descriptive Name"="Protocol LIN Frame Checksum Value", "Data Type"=0, "Command"="BUS{SerialBus}:LIN:FRAM<Frame>:CSV?", 
